vi "microspec_validating.vi"() -> ()   [LabVIEW 2009]
uses:
  <vilib>/Utility/file.llb/Write To Spreadsheet File (string).vi
  <vilib>/Instr/_visa.llb/VISA Configure Serial Port (Instr).vi
panel:
  out "error 2":dbl
  in  "Path":path
  in  "intergration time":dbl caption="sensor\nintergration time (us)" min=54.0 max=5000000.0 step=100.0
  in  "?":T1(tab)
  out "radiometer data file path":path
  in  "Runname":string
  out "Sensor_name":string
  out "Radiometer Average":dbl
  in  "Delay":dbl
  in  "Step":dbl
  in  "Stop Wl":dbl min=0.0 max=5000.0 step=100.0
  in  "Start Wl":dbl min=0.0 max=5000.0 step=100.0
  in  "mean_number":i32 caption="Mean Number"
  out "Current Wavelength":dbl
  out "XY-Graph 2":cluster{"Y":dbl[], "Y":dbl[]}[](graph)
  in  "run 5":bool
  out "sectrometer data file path":path
  in  "save data":bool
  in  "reset with every wavelength?":bool caption="reset with new run?"
  in  "Delay":dbl
  in  "Step":dbl
  in  "Stop Wl":dbl min=0.0 max=5000.0 step=100.0
  out "Current Wavelength":dbl
  in  "Start Wl 2":dbl min=0.0 max=5000.0 step=10.0
  in  "Sensor":string(combo)
  in  "run 2":bool
  in  "Set Runs":i32
  out "Current Run":i32
  in  "stop runs":bool
  out "raw_data":cluster{"Y":dbl[], "Y":dbl[]}[](graph) caption="raw data"
  out "error":dbl
  out "raw_data 2":cluster{"Y":dbl[], "Y":dbl[]}[](graph) caption="raw data"
  in  "Stopp":bool
  out "System Setup":i32
  out "DLL Version":string
  out "Get Version":i32
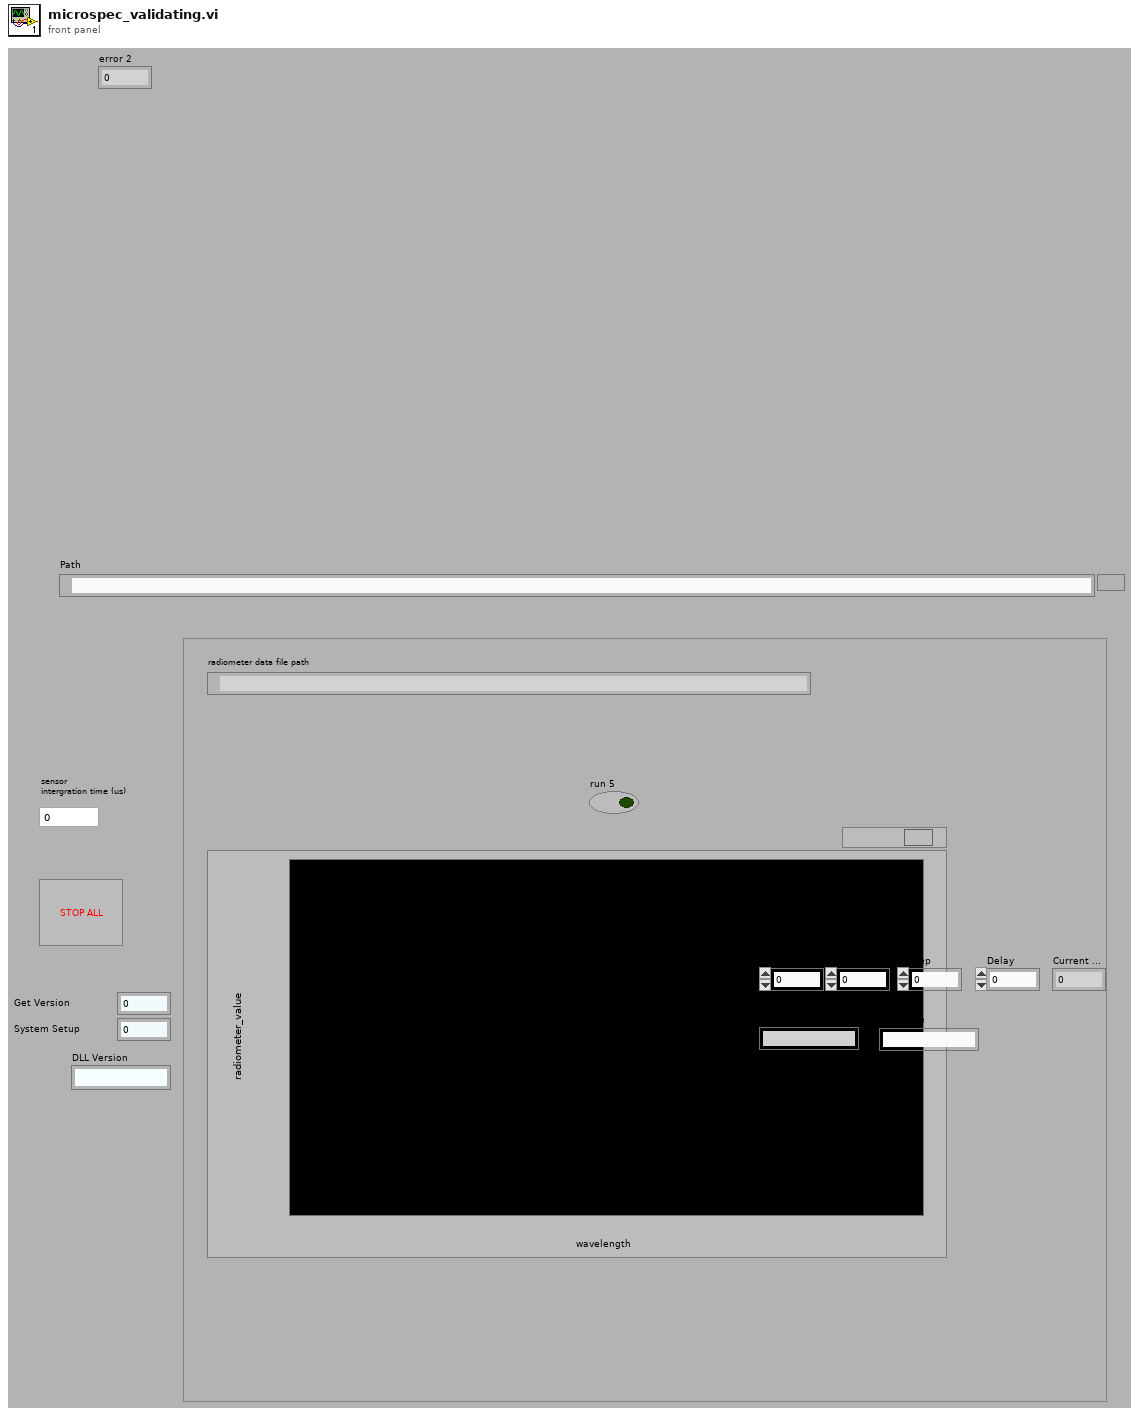
[diagram p1: front panel]
types:
  T1 = enum32{"radiometer calibration", "measuring sequence", "microspec standalone"}
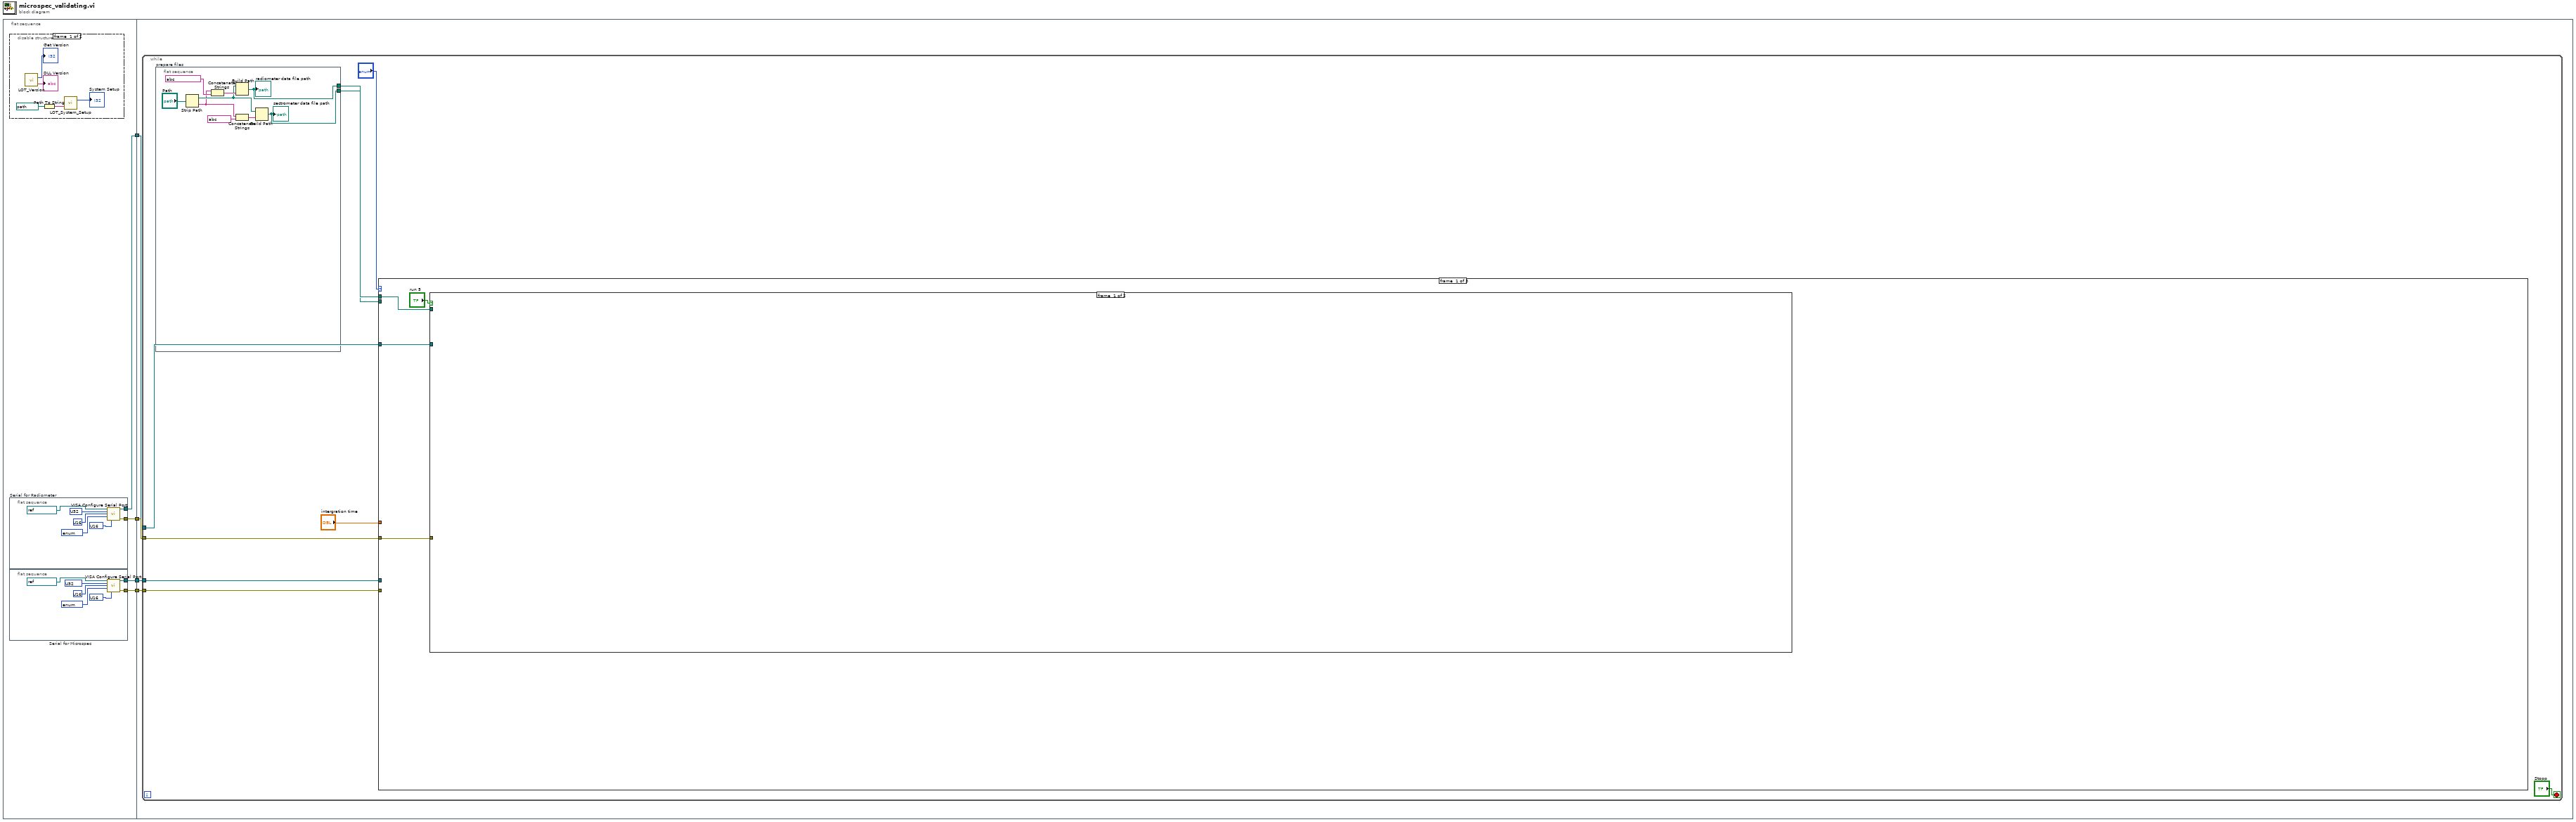
[diagram p0: block diagram]
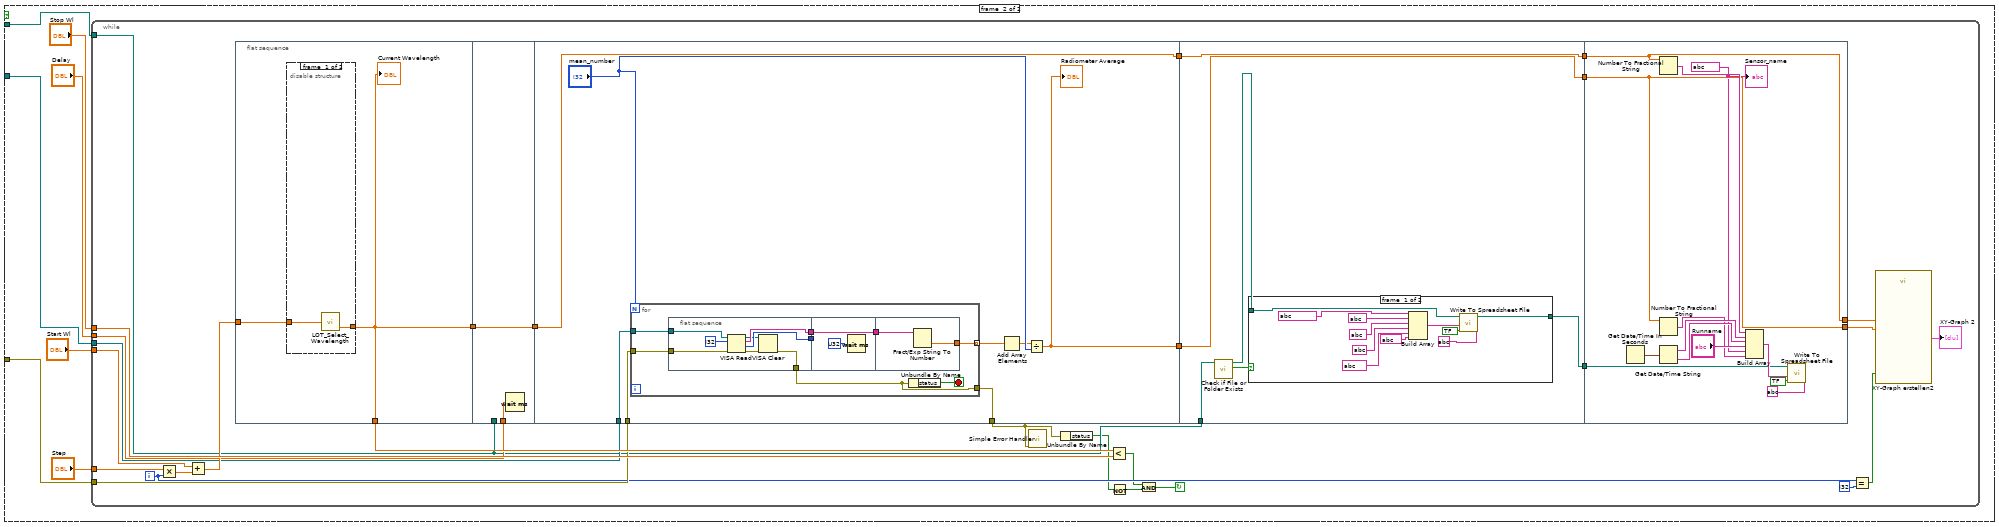
[diagram p3: hidden frame]
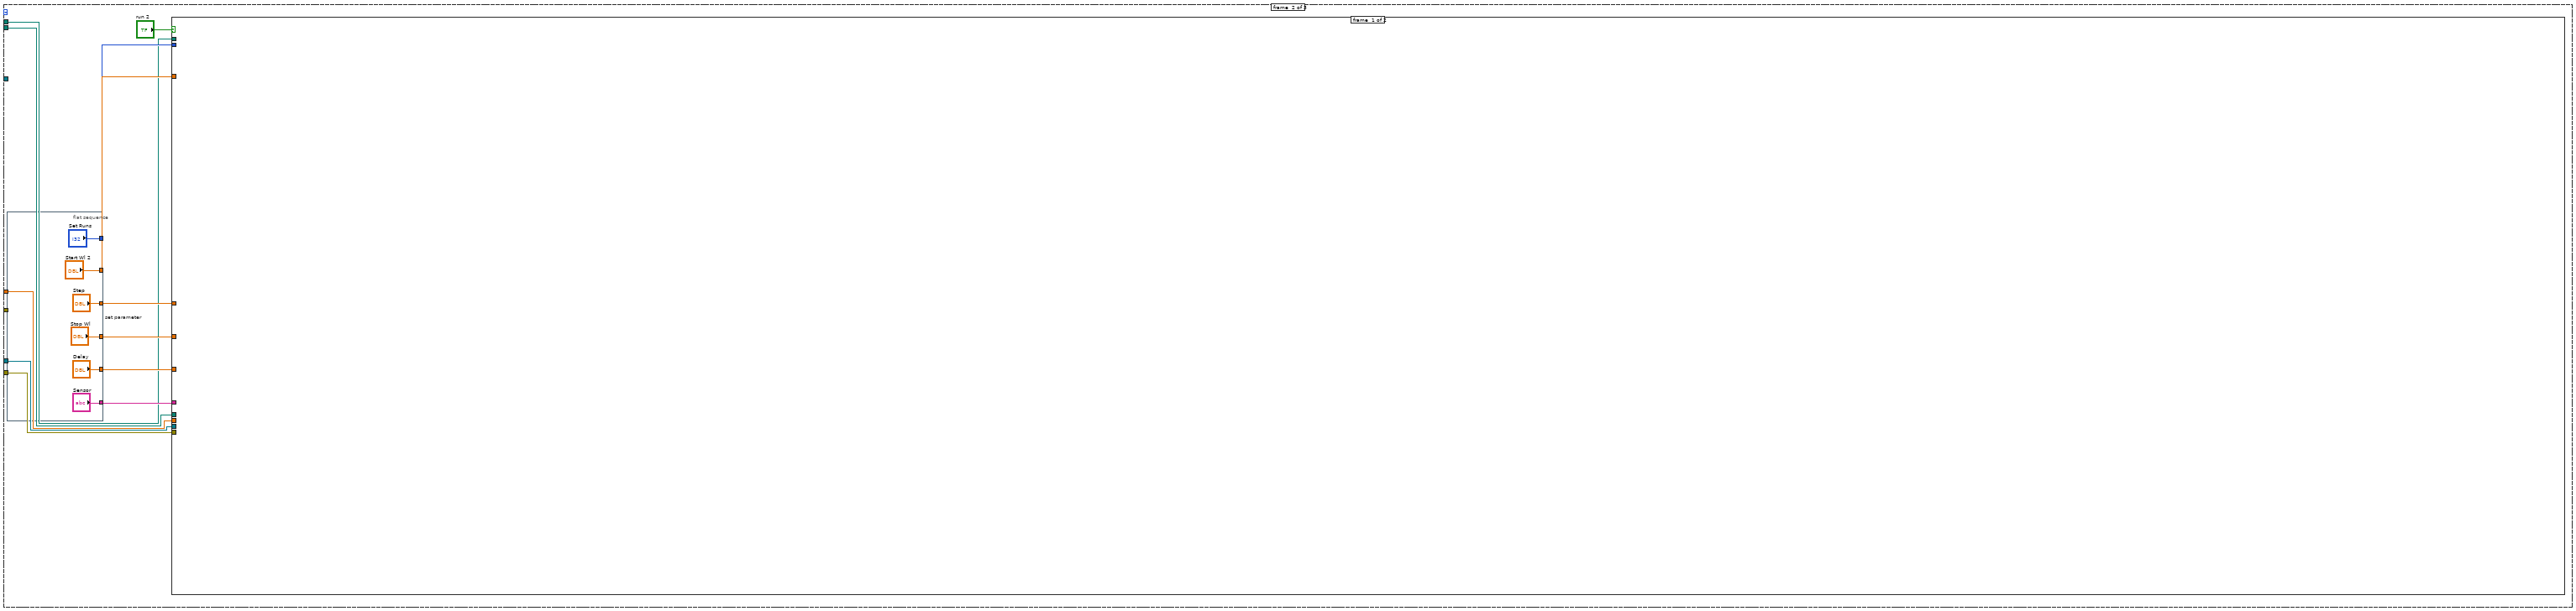
[diagram p6: hidden frame]
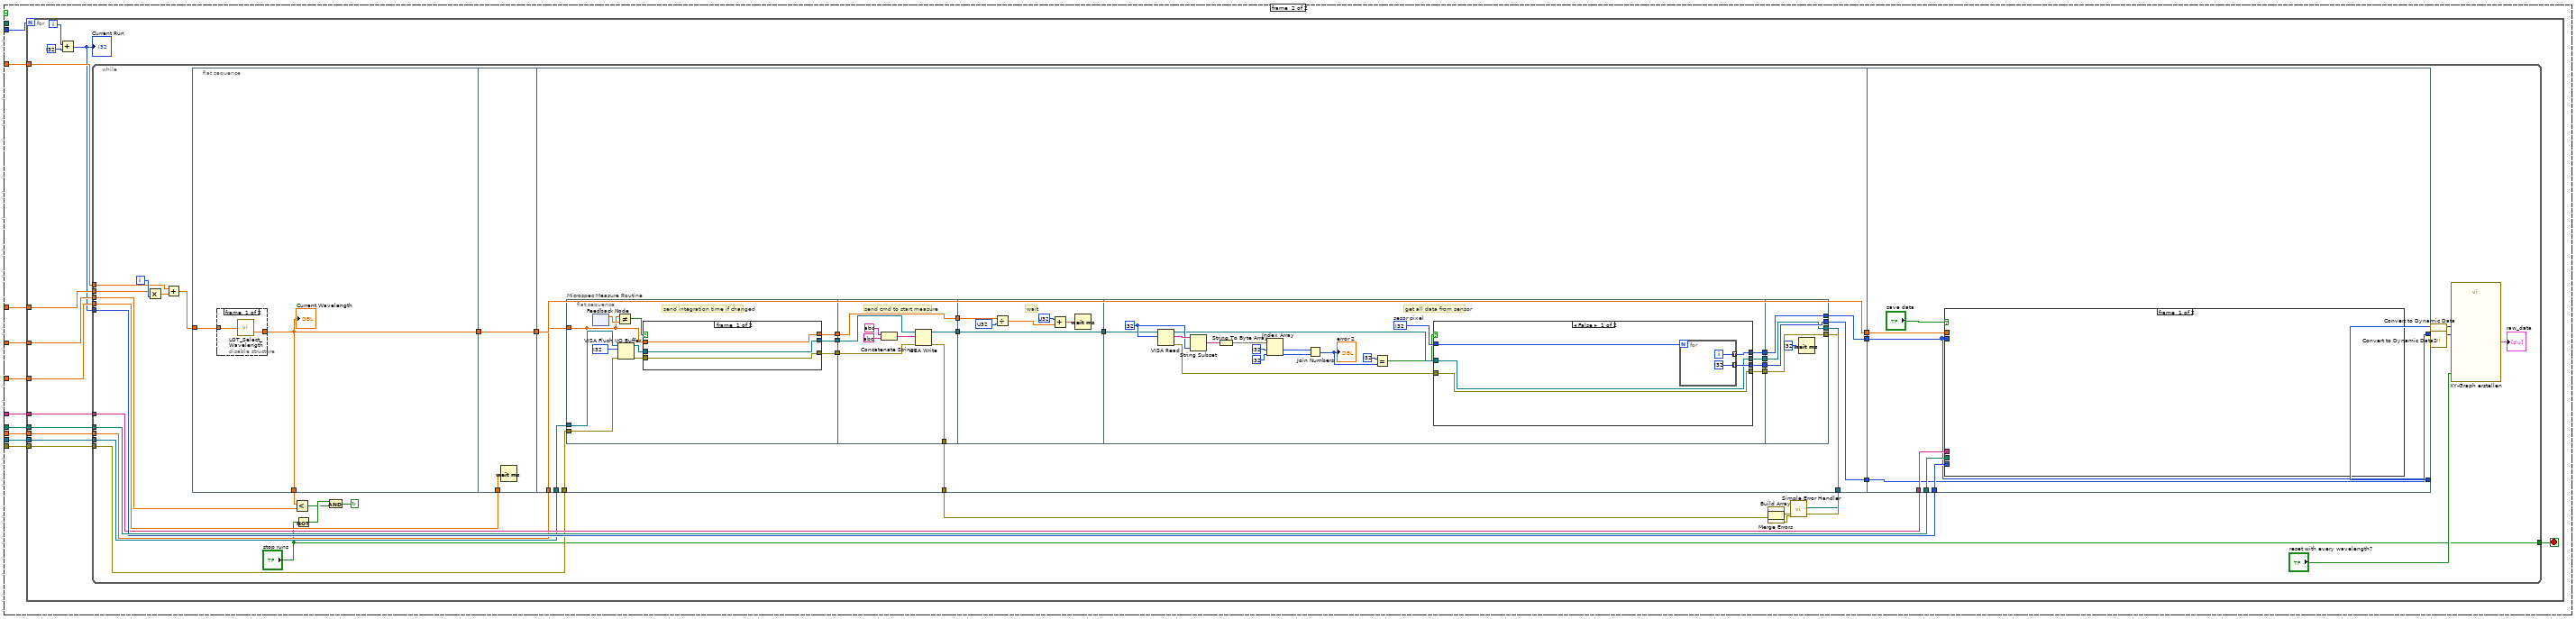
[diagram p7: hidden frame]
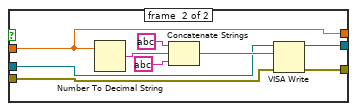
[diagram p9: hidden frame]
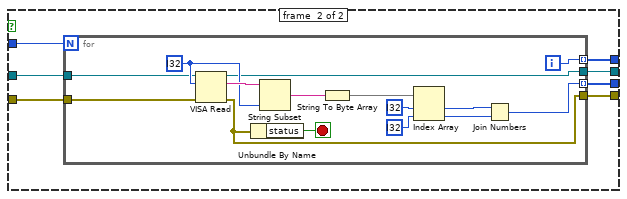
[diagram p10: hidden frame]
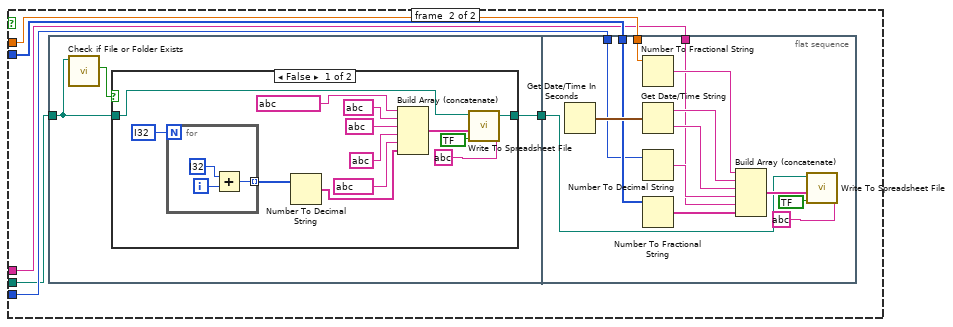
[diagram p11: hidden frame]
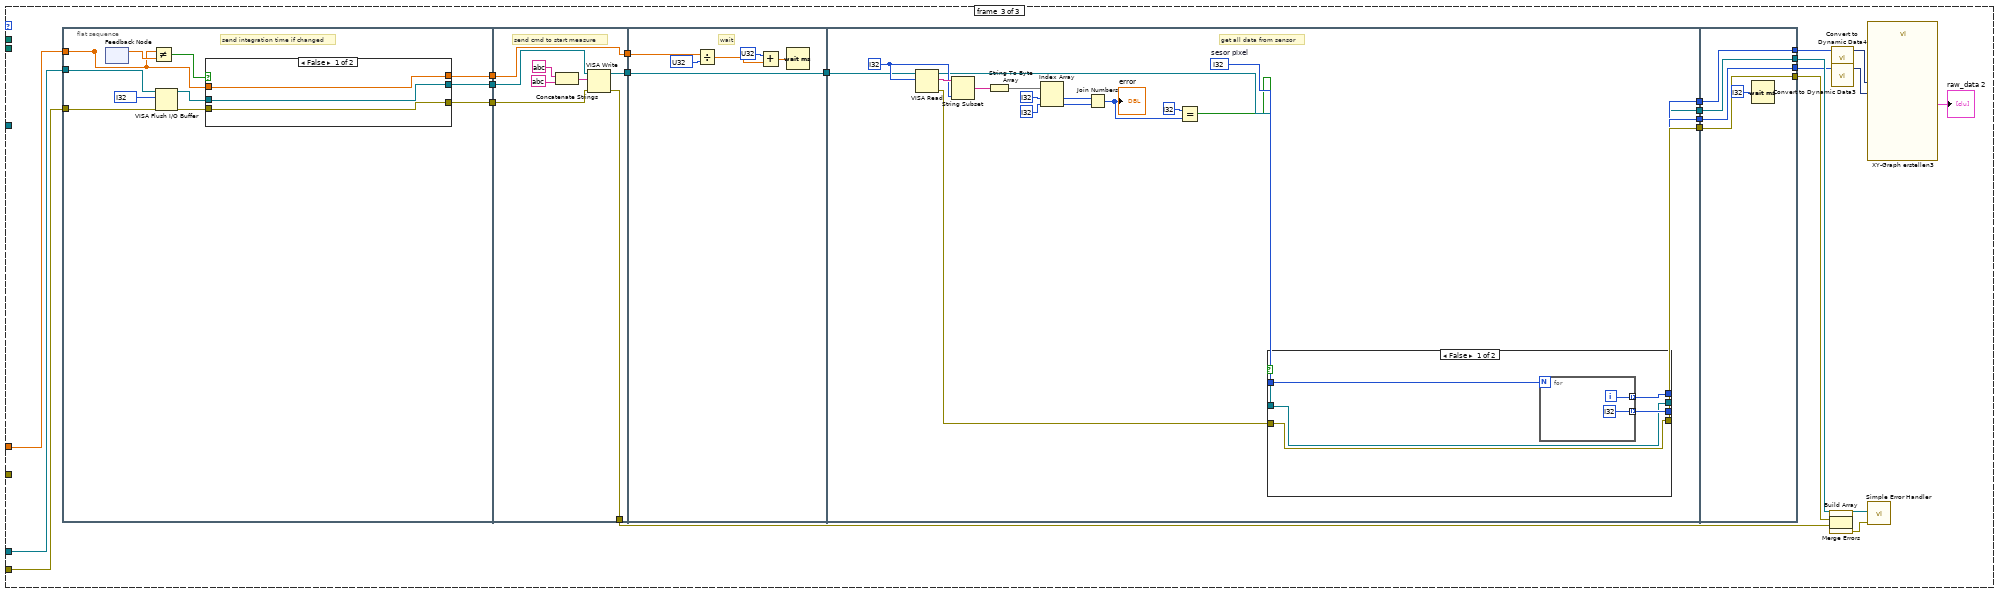
[diagram p13: hidden frame]
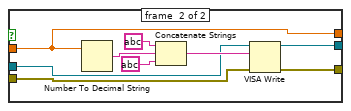
[diagram p14: hidden frame]
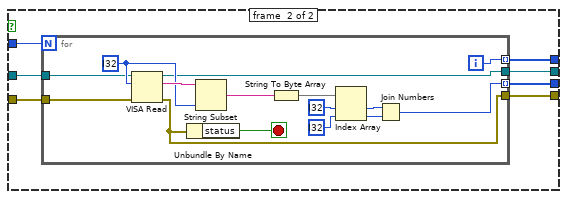
[diagram p15: hidden frame]
diagram:
  n1 = flat-sequence {
    tunnel: [w8] -> w4
    tunnel: [w7] -> w3
    tunnel: [w6] -> w2
    tunnel: [w5] -> w1
    tunnel: w4 -> [w31]
    tunnel: w3 -> [w30]
    tunnel: w2 -> [w29]
    tunnel: w1 -> [w28]
    frame #0 {
      # "Configuration"
      n2 = disable-structure shown="Enabled" {
        frame #0 {
          n3 = call "LOT_Version.vi"() -> ("Version"=→"DLL Version":string, "Get Version"=→"Get Version":i32)
          n4 = Path To String(path=path ? ("Configuration File")) -> (string=w25:string)
          n5 = call "LOT_System_Setup.vi"("CFG File Path"=w25) -> ("Error Code"=→"System Setup":i32)  [unwired: 2 in]
        }
        frame #1 {
        }
      }
      n6 = flat-sequence "Serial for Radiometer" {
        tunnel: [w15] -> w6
        tunnel: [w14] -> w5
        frame #0 {
          w10 = u16 ? items=["1.0", "1.5", "2.0"] ("stop bits (10: 1 bit)")
          n7 = call-poly "VISA Configure Serial Port"("VISA resource name"=refnum<visa-resource-name> ?, "baud rate (9600)"=u32 ?, "data bits (8)"=u16 ?, "parity (0:none)"=enum16{"None", "Odd", "Even", "Mark", "Space"} ?, "stop bits (10: 1 bit)"=w10) -> ("VISA resource name out"=w14:refnum<visa-resource-name>, "error out"=w15:errorcluster)  [unwired: 9 in]
        }
      }
      n8 = flat-sequence "Serial for Microspec" {
        tunnel: [w22] -> w8
        tunnel: [w21] -> w7
        frame #0 {
          w17 = u16 ? items=["1.0", "1.5", "2.0"] ("stop bits (10: 1 bit)")
          n9 = call-poly "VISA Configure Serial Port"("VISA resource name"=refnum<visa-resource-name> ?, "baud rate (9600)"=u32 ?, "data bits (8)"=u16 ?, "parity (0:none)"=enum16{"None", "Odd", "Even", "Mark", "Space"} ?, "stop bits (10: 1 bit)"=w17) -> ("VISA resource name out"=w22:refnum<visa-resource-name>, "error out"=w21:errorcluster)  [unwired: 9 in]
        }
      }
    }
    frame #1 {
      n10 = while {
        tunnel: w31 -> [w38]
        tunnel: w30 -> [w37]
        tunnel: w29 -> [w36]
        tunnel: w28 -> [w35]
        stop <- "Stopp" stop-if-true
        n11 = flat-sequence "prepare files" {
          tunnel: [w41] -> w32
          tunnel: [w42] -> w33
          frame #0 {
            n12 = Strip Path(path="Path") -> (stripped path=w44:path, name=w43:string)
            n13 = Concatenate Strings(w43, string ?) -> (w45:string)
            n14 = Build Path(base path=w44, name or relative path=w45) -> (appended path=w42:path)
            "radiometer data file path" <- w42
            n15 = Concatenate Strings(w43, string ?) -> (w47:string)
            n16 = Build Path(base path=w44, name or relative path=w47) -> (appended path=w41:path)
            "sectrometer data file path" <- w41
          }
        }
        n17 = case shown="\"measuring sequence\"" "?" {
          tunnel: w32 -> [_ w165 _]
          tunnel: w38 -> [_ w164 w415]
          tunnel: w37 -> [_ w163 w414]
          tunnel: w36 -> [w52 _ _]
          tunnel: w35 -> [w51 _ _]
          tunnel: "intergration time" -> [_ w162 w413]
          tunnel: w33 -> [w50 w155 _]
          frame #0 {
            n18 = case shown="True" "run 5" {
              tunnel: w50 -> [_ w56]
              tunnel: w52 -> [_ w55]
              tunnel: w51 -> [_ w54]
              frame #0 {
              }
              frame #1 {
                n19 = while {
                  tunnel: "Step" -> [w88]
                  tunnel: "Start Wl" -> [w86]
                  tunnel: "Stop Wl" -> [w85]
                  tunnel: "Delay" -> [w81]
                  tunnel: w56 -> [w67]
                  tunnel: w54 -> [w80]
                  tunnel: w55 -> [w79]
                  i -> [w75]
                  stop <- w62 continue-if-true
                  n20 = Multiply(x=w88, y=w75) -> (x*y=w87:dbl)
                  n21 = Add(x=w86, y=w87) -> (x+y=w84:dbl)
                  n22 = flat-sequence {
                    tunnel: w84 -> [w90]
                    tunnel: [w89] -> w83
                    tunnel: [w89] -> w82
                    tunnel: w67 -> [_]
                    tunnel: w82 -> [w94]
                    tunnel: w81 -> [w95]
                    tunnel: [w94] -> w78
                    tunnel: w80 -> [w103]
                    tunnel: w79 -> [w102]
                    tunnel: w78 -> [w101]
                    tunnel: [w101] -> w71
                    tunnel: [w99] -> w69
                    tunnel: [w96] -> w61
                    tunnel: w71 -> [w129]
                    tunnel: [w129] -> w70
                    tunnel: w69 -> [w128]
                    tunnel: [w128] -> w68
                    tunnel: w67 -> [w126]
                    tunnel: [w127] -> w66
                    tunnel: [w145] -> w72
                    tunnel: [w146] -> w76
                    tunnel: w70 -> [w146]
                    tunnel: w68 -> [w145]
                    tunnel: w66 -> [w148]
                    frame #0 {
                      n23 = disable-structure shown="Enabled" {
                        disable-tunnel: w90 -> [w92 w93]
                        disable-tunnel: [w91 w93] -> w89
                        frame #0 {
                          n24 = call "LOT_Select_Wavelength.vi"("Input Wavelength"=w92) -> ("Current Wavelength"=w91:dbl)  [unwired: 1 out]
                        }
                        frame #1 {
                        }
                      }
                      "Current Wavelength" <- w89
                    }
                    frame #1 {
                      n25 = Wait (ms)(milliseconds to wait=w95) -> ()  [unwired: 1 out]
                    }
                    frame #2 {
                      n26 = for {
                        N: "mean_number" -> [_]
                        tunnel: w103 -> [w108]
                        tunnel: w102 -> [w107]
                        tunnel: [w106] -> w97 mode=indexing
                        tunnel: [w105] -> w96
                        stop <- w104 stop-if-true
                        n27 = flat-sequence {
                          tunnel: [w116] -> w111
                          tunnel: w108 -> [w119]
                          tunnel: w107 -> [w118]
                          tunnel: [w115] -> w110
                          tunnel: [w112] -> w105
                          tunnel: w111 -> [w121]
                          tunnel: [w121] -> w109
                          tunnel: w110 -> [_]
                          tunnel: w109 -> [w122]
                          tunnel: [w123] -> w106
                          frame #0 {
                            n28 = VISA Read(VISA resource name=w119, byte count=i32 ?, error in (no error)=w118) -> (VISA resource name out=w113:refnum<visa-resource-name>, read buffer=w116:string, return count=w115:u32, error out=w114:errorcluster)
                            n29 = VISA Clear(VISA resource name=w113, error in (no error)=w114) -> (error out=w112:errorcluster)  [unwired: 1 out]
                          }
                          frame #1 {
                            n30 = Wait (ms)(milliseconds to wait=u32 ? ("Zu wartende ms")) -> ()  [unwired: 1 out]
                          }
                          frame #2 {
                            n31 = Fract/Exp String To Number(string=w122) -> (number=w123:dbl)  [unwired: 3 in, 1 out]
                          }
                        }
                        n32 = Unbundle By Name(w105) -> ("status"=w104:bool)
                      }
                      n33 = Add Array Elements(numeric array=w97) -> (sum=w98:dbl)
                      n34 = Divide(x=w98, y="mean_number") -> (x/y=w99:dbl)
                      "Radiometer Average" <- w99
                    }
                    frame #3 {
                      n35 = call <vilib>:"Check if File or Folder Exists.vi"("path"=w126) -> ("file or folder exists?"=w125:bool, "dup path"=w124:path)  [unwired: 8 in, 1 out]
                      n36 = case shown="True" w125 {
                        tunnel: w124 -> [w138 w141]
                        tunnel: [w131 w141] -> w127
                        frame #0 {
                          n37 = Build Array(string ?, string ? ("Element"), string ? ("Element"), string ? ("Element"), string ? ("Element"), string ?) -> (w140:string[])
                          n38 = call-poly <vilib>:"Write To Spreadsheet File.vi"("delimiter (\\t)"=string ?, "append to file? (new file:F)"=bool ?, "1D data"=w140, "file path (dialog if empty)"=w138) -> ("new file path (Not A Path if cancelled)"=w131:path)  [unwired: 4 in]
                        }
                        frame #1 {
                        }
                      }
                    }
                    frame #4 {
                      w143 = string ? ("Sensor_name")
                      n39 = Get Date/Time In Seconds() -> (seconds since 1Jan1904=w153:timestamp)
                      n40 = Number To Fractional String(number=w146) -> (F-format string=w154:string)  [unwired: 3 in]
                      n41 = Number To Fractional String(number=w145) -> (F-format string=w142:string)  [unwired: 3 in]
                      n42 = Get Date/Time String(seconds (now)=w153) -> (date string=w152:string, time string=w151:string)  [unwired: 2 in]
                      n43 = Build Array(w154, w152, w151, "Runname", w143, w142) -> (w150:string[])
                      n44 = call-poly <vilib>:"Write To Spreadsheet File.vi"("delimiter (\\t)"=string ?, "append to file? (new file:F)"=bool ?, "1D data"=w150, "file path (dialog if empty)"=w148) -> ()  [unwired: 4 in, 1 out]
                      "Sensor_name" <- w143
                    }
                  }
                  n45 = call <vilib>:"Simple Error Handler.vi"("error in (no error)"=w61) -> ()  [unwired: 4 in, 5 out]
                  n46 = Unbundle By Name(w61) -> ("status"=w63:bool)
                  n47 = Less?(x=w83, y=w85) -> (x < y?=w65:bool)
                  n48 = Not(x=w63) -> (.not. x?=w64:bool)
                  n49 = And(x=w65, y=w64) -> (x .and. y?=w62:bool)
                  n50 = Equal?(x=w75, y=i32 ?) -> (x = y?=w73:bool)
                  n51 = call "XY-Graph erstellen2"("Reset"=w73, "Y Input"=w72, "X Input"=w76) -> ("XY Graph"=→"XY-Graph 2":cluster{"Y":dbl[], "Y":dbl[]}[])  [unwired: 7 in, 1 out]
                }
              }
            }
          }
          frame #1 {
            n52 = flat-sequence "set parameter" {
              tunnel: ["Sensor"] -> w161
              tunnel: ["Delay"] -> w160
              tunnel: ["Step"] -> w159
              tunnel: ["Stop Wl"] -> w158
              tunnel: ["Start Wl 2"] -> w157
              tunnel: ["Set Runs"] -> w156
              frame #0 {
              }
            }
            n53 = case shown="True" "run 2" {
              tunnel: w165 -> [_ w173]
              tunnel: w161 -> [_ w182]
              tunnel: w156 -> [_ w181]
              tunnel: w164 -> [_ w180]
              tunnel: w163 -> [_ w179]
              tunnel: w160 -> [_ w178]
              tunnel: w158 -> [_ w177]
              tunnel: w159 -> [_ w176]
              tunnel: w157 -> [_ w175]
              tunnel: w162 -> [_ w174]
              tunnel: w155 -> [_ _]
              frame #0 {
              }
              frame #1 {
                n54 = for {
                  N: w181 -> [_]
                  tunnel: w173 -> [w195]
                  tunnel: w182 -> [w194]
                  tunnel: w180 -> [w193]
                  tunnel: w179 -> [w192]
                  tunnel: w178 -> [w191]
                  tunnel: w177 -> [w190]
                  tunnel: w176 -> [w189]
                  tunnel: w175 -> [w188]
                  tunnel: w174 -> [w187]
                  i -> [w186]
                  stop <- w183 stop-if-true
                  n55 = Add(x=w186, y=i32 ?) -> (x+y=w185:i32)
                  "Current Run" <- w185
                  n56 = while {
                    tunnel: w195 -> [w227]
                    tunnel: w185 -> [w226]
                    tunnel: w194 -> [w222]
                    tunnel: w193 -> [w220]
                    tunnel: w192 -> [w219]
                    tunnel: w191 -> [w210]
                    tunnel: w190 -> [w208]
                    tunnel: w189 -> [w207]
                    tunnel: w188 -> [w206]
                    tunnel: w187 -> [w205]
                    tunnel: ["stop runs"] -> w183
                    i -> [w224]
                    stop <- w199 continue-if-true
                    n57 = Multiply(x=w207, y=w224) -> (x*y=w229:dbl)
                    n58 = Add(x=w206, y=w229) -> (x+y=w228:dbl)
                    n59 = flat-sequence {
                      tunnel: w228 -> [w231]
                      tunnel: [w230] -> w225
                      tunnel: [w230] -> w209
                      tunnel: w225 -> [w235]
                      tunnel: w210 -> [w236]
                      tunnel: [w235] -> w213
                      tunnel: [w244] -> w221
                      tunnel: w220 -> [w248]
                      tunnel: w219 -> [w249]
                      tunnel: [w247] -> w217
                      tunnel: [w246] -> w216
                      tunnel: [w245] -> w215
                      tunnel: w213 -> [w244]
                      tunnel: w205 -> [w243]
                      tunnel: [w242] -> w204
                      tunnel: [w241] -> w197
                      tunnel: w227 -> [w352]
                      tunnel: w221 -> [w351]
                      tunnel: w226 -> [w350]
                      tunnel: [w348] -> w211
                      tunnel: w222 -> [w349]
                      tunnel: w215 -> [w348]
                      tunnel: w204 -> [w347]
                      tunnel: [w347] -> w203
                      frame #0 {
                        # "set wavelength"
                        n60 = disable-structure shown="Enabled" {
                          disable-tunnel: w231 -> [w233 w234]
                          disable-tunnel: [w232 w234] -> w230
                          frame #0 {
                            n61 = call "LOT_Select_Wavelength.vi"("Input Wavelength"=w233) -> ("Current Wavelength"=w232:dbl)  [unwired: 1 out]
                          }
                          frame #1 {
                          }
                        }
                        "Current Wavelength" <- w230
                      }
                      frame #1 {
                        # "wait"
                        n62 = Wait (ms)(milliseconds to wait=w236) -> ()  [unwired: 1 out]
                      }
                      frame #2 {
                        n63 = flat-sequence "Microspec Measure Routine" {
                          tunnel: w248 -> [w257]
                          tunnel: w249 -> [w266]
                          tunnel: [w261] -> w255
                          tunnel: [w260] -> w254
                          tunnel: [w259] -> w253
                          tunnel: w243 -> [w256]
                          tunnel: [w283] -> w252
                          tunnel: [w282] -> w246
                          tunnel: w255 -> [w280]
                          tunnel: w254 -> [w281]
                          tunnel: w253 -> [w279]
                          tunnel: [w279] -> w251
                          tunnel: w252 -> [w288]
                          tunnel: [w288] -> w250
                          tunnel: w251 -> [w287]
                          tunnel: w250 -> [w297]
                          tunnel: [w296] -> w240
                          tunnel: [w295] -> w239
                          tunnel: [w294] -> w238
                          tunnel: [w293] -> w237
                          tunnel: [w342] -> w241
                          tunnel: [w343] -> w247
                          tunnel: [w344] -> w242
                          tunnel: [w345] -> w245
                          tunnel: w240 -> [w345]
                          tunnel: w239 -> [w344]
                          tunnel: w238 -> [w343]
                          tunnel: w237 -> [w342]
                          frame #0 {
                            # "send integration time if changed"
                            n64 = feedback #1() -> (w265:dbl)  [unwired: 1 in]
                            n65 = Not Equal?(x=w256, y=w265) -> (x != y?=w264:bool)
                            n66 = VISA Flush I/O Buffer(VISA resource name=w257, mask (16)=i32 ?, error in (no error)=w266) -> (VISA resource name out=w263:refnum<visa-resource-name>, error out=w262:errorcluster)
                            n67 = case shown="True" w264 {
                              tunnel: w263 -> [w268 w274]
                              tunnel: w262 -> [w267 w273]
                              tunnel: [w267 w272] -> w261
                              tunnel: [w268 w271] -> w260
                              tunnel: w256 -> [w269 w270]
                              tunnel: [w269 w270] -> w259
                              frame #0 {
                              }
                              frame #1 {
                                n68 = Number To Decimal String(number=w270) -> (decimal integer string=w277:string)  [unwired: 1 in]
                                n69 = Concatenate Strings(string ?, w277, string ?) -> (w275:string)
                                n70 = VISA Write(VISA resource name=w274, write buffer=w275, error in (no error)=w273) -> (VISA resource name out=w271:refnum<visa-resource-name>, error out=w272:errorcluster)  [unwired: 1 out]
                              }
                            }
                          }
                          frame #1 {
                            # "send cmd to start measure"
                            n71 = Concatenate Strings(string ?, string ?) -> (w284:string)
                            n72 = VISA Write(VISA resource name=w281, write buffer=w284, error in (no error)=w280) -> (VISA resource name out=w283:refnum<visa-resource-name>, error out=w282:errorcluster)  [unwired: 1 out]
                          }
                          frame #2 {
                            # "wait"
                            n73 = Divide(x=w287, y=u32 ? ("Zu wartende ms")) -> (x/y=w289:dbl)
                            n74 = Add(x=u32 ? ("Zu wartende ms"), y=w289) -> (x+y=w291:dbl)
                            n75 = Wait (ms)(milliseconds to wait=w291) -> ()  [unwired: 1 out]
                          }
                          frame #3 {
                            w309 = i32 ?
                            w311 = i32 ?  # sesor pixel
                            # "get all data from sensor"
                            n76 = VISA Read(VISA resource name=w297, byte count=w309) -> (VISA resource name out=w302:refnum<visa-resource-name>, read buffer=w310:string, error out=w299:errorcluster)  [unwired: 1 in, 1 out]
                            n77 = String Subset(string=w310, length (rest)=w309) -> (substring=w308:string)  [unwired: 1 in]
                            n78 = String To Byte Array(string=w308) -> (unsigned byte array=w307:u8[])
                            n79 = Index Array(array=w307, index #1=i32 ?, index #2=i32 ?) -> (element #1=w303:u8, element #2=w304:u8)
                            n80 = Join Numbers(hi=w303, lo=w304) -> ((hi.lo)=w300:u16)
                            "error 2" <- w300
                            n81 = Equal?(x=i32 ?, y=w300) -> (x = y?=w298:bool)
                            n82 = case shown="False" w298 {
                              tunnel: [w314 w325] -> w294
                              tunnel: w302 -> [w313 w324]
                              tunnel: [w315 w323] -> w295
                              tunnel: [w316 w322] -> w296
                              tunnel: w311 -> [w312 w321]
                              tunnel: [w313 w320] -> w293
                              tunnel: w299 -> [w314 w319]
                              frame #0 {
                                n83 = for {
                                N: w312 -> [_]
                                tunnel: [i32 ?] -> w315 mode=indexing
                                tunnel: [w318] -> w316 mode=indexing
                                i -> [w318]
                                }
                              }
                              frame #1 {
                                n84 = for {
                                N: w321 -> [_]
                                tunnel: w324 -> [w330]
                                tunnel: [w329] -> w325
                                tunnel: [w332] -> w323 mode=indexing
                                tunnel: [w331] -> w322 mode=indexing
                                tunnel: [w327] -> w320
                                tunnel: w319 -> [w326]
                                i -> [w331]
                                stop <- w328 stop-if-true
                                w339 = i32 ?
                                n85 = VISA Read(VISA resource name=w330, byte count=w339, error in (no error)=w326) -> (VISA resource name out=w327:refnum<visa-resource-name>, read buffer=w340:string, error out=w329:errorcluster)  [unwired: 1 out]
                                n86 = Unbundle By Name(w329) -> ("status"=w328:bool)
                                n87 = String Subset(string=w340, length (rest)=w339) -> (substring=w338:string)  [unwired: 1 in]
                                n88 = String To Byte Array(string=w338) -> (unsigned byte array=w337:u8[])
                                n89 = Index Array(array=w337, index #1=i32 ?, index #2=i32 ?) -> (element #1=w333:u8, element #2=w334:u8)
                                n90 = Join Numbers(hi=w333, lo=w334) -> ((hi.lo)=w332:u16)
                                }
                              }
                            }
                          }
                          frame #4 {
                            n91 = Wait (ms)(milliseconds to wait=i32 ?) -> ()  [unwired: 1 out]
                          }
                        }
                      }
                      frame #3 {
                        n92 = case shown="True" "save data" {
                          tunnel: w352 -> [_ w355]
                          tunnel: w351 -> [_ w357]
                          tunnel: w350 -> [_ w356]
                          tunnel: w348 -> [_ w358]
                          tunnel: w349 -> [_ w354]
                          frame #0 {
                          }
                          frame #1 {
                            n93 = flat-sequence {
                              tunnel: w355 -> [w361]
                              tunnel: [w359] -> w353
                              tunnel: w358 -> [w385]
                              tunnel: w357 -> [w384]
                              tunnel: w356 -> [w383]
                              tunnel: w354 -> [w381]
                              tunnel: w353 -> [w379]
                              frame #0 {
                                n94 = call <vilib>:"Check if File or Folder Exists.vi"("path"=w361) -> ("file or folder exists?"=w360:bool)  [unwired: 8 in, 2 out]
                                n95 = case shown="False" w360 {
                                tunnel: w361 -> [w365 w378]
                                tunnel: [w362 w378] -> w359
                                frame #0 {
                                n96 = for {
                                N: i32 ? -> [_]
                                tunnel: [w375] -> w368 mode=indexing
                                i -> [w377]
                                n97 = Add(x=i32 ?, y=w377) -> (x+y=w375:i32)
                                }
                                n98 = Number To Decimal String(number=w368) -> (decimal integer string=w370:string[])  [unwired: 1 in]
                                n99 = Build Array (concatenate)(string ?, string ? ("Element"), string ? ("Element"), string ? ("Element"), string ? ("Element"), w370) -> (w374:string[])
                                n100 = call-poly <vilib>:"Write To Spreadsheet File.vi"("delimiter (\\t)"=string ?, "append to file? (new file:F)"=bool ?, "1D data"=w374, "file path (dialog if empty)"=w365) -> ("new file path (Not A Path if cancelled)"=w362:path)  [unwired: 4 in]
                                }
                                frame #1 {
                                }
                                }
                              }
                              frame #1 {
                                n101 = Get Date/Time In Seconds() -> (seconds since 1Jan1904=w387:timestamp)
                                n102 = Number To Fractional String(number=w384) -> (F-format string=w386:string)  [unwired: 3 in]
                                n103 = Get Date/Time String(seconds (now)=w387) -> (date string=w388:string, time string=w389:string)  [unwired: 2 in]
                                n104 = Number To Decimal String(number=w383) -> (decimal integer string=w382:string)  [unwired: 1 in]
                                n105 = Number To Fractional String(number=w385) -> (F-format string=w392:string[])  [unwired: 3 in]
                                n106 = Build Array (concatenate)(w386, w388, w389, w382, w381, w392) -> (w390:string[])
                                n107 = call-poly <vilib>:"Write To Spreadsheet File.vi"("delimiter (\\t)"=string ?, "append to file? (new file:F)"=bool ?, "1D data"=w390, "file path (dialog if empty)"=w379) -> ()  [unwired: 4 in, 1 out]
                              }
                            }
                          }
                        }
                      }
                    }
                    n108 = Less?(x=w209, y=w208) -> (x < y?=w200:bool)
                    n109 = Not(x="stop runs") -> (.not. x?=w201:bool)
                    n110 = And(x=w201, y=w200) -> (x .and. y?=w199:bool)
                    n111 = Build Array(w217, w216) -> (w196:errorcluster[])
                    n112 = call <vilib>:"Merge Errors.vi"("error array in"=w196) -> ("error out"=w218:errorcluster)  [unwired: 6 in]
                    n113 = call <vilib>:"Simple Error Handler.vi"("error source (\" \")"=w197, "error in (no error)"=w218) -> ()  [unwired: 3 in, 5 out]
                    n114 = call "Convert to Dynamic Data"("Array"=w203) -> ("Dynamic Data Type"=w212:dynamicdata)  [unwired: 3 in]
                    n115 = call "Convert to Dynamic Data2"("Array"=w211) -> ("Dynamic Data Type"=w214:dynamicdata)  [unwired: 3 in]
                    n116 = call "XY-Graph erstellen"("Reset"="reset with every wavelength?", "Y Input"=w214, "X Input"=w212) -> ("XY Graph"=→"raw_data":cluster{"Y":dbl[], "Y":dbl[]}[])  [unwired: 7 in, 1 out]
                  }
                }
              }
            }
          }
          frame #2 {
            n117 = flat-sequence {
              tunnel: w415 -> [w425]
              tunnel: w414 -> [w426]
              tunnel: [w420] -> w412
              tunnel: [w419] -> w411
              tunnel: [w418] -> w410
              tunnel: w413 -> [w416]
              tunnel: [w443] -> w409
              tunnel: [w442] -> w405
              tunnel: w412 -> [w440]
              tunnel: w411 -> [w441]
              tunnel: w410 -> [w439]
              tunnel: [w439] -> w408
              tunnel: w409 -> [w448]
              tunnel: [w448] -> w407
              tunnel: w408 -> [w447]
              tunnel: w407 -> [w458]
              tunnel: [w471] -> w397
              tunnel: [w470] -> w396
              tunnel: [w469] -> w395
              tunnel: [w467] -> w394
              tunnel: [w502] -> w403
              tunnel: [w503] -> w398
              tunnel: [w504] -> w399
              tunnel: [w505] -> w406
              tunnel: w397 -> [w505]
              tunnel: w396 -> [w504]
              tunnel: w395 -> [w503]
              tunnel: w394 -> [w502]
              frame #0 {
                # "send integration time if changed"
                n118 = feedback #2() -> (w424:dbl)  [unwired: 1 in]
                n119 = Not Equal?(x=w416, y=w424) -> (x != y?=w423:bool)
                n120 = VISA Flush I/O Buffer(VISA resource name=w425, mask (16)=i32 ?, error in (no error)=w426) -> (VISA resource name out=w422:refnum<visa-resource-name>, error out=w421:errorcluster)
                n121 = case shown="False" w423 {
                  tunnel: w422 -> [w428 w434]
                  tunnel: w421 -> [w427 w433]
                  tunnel: [w427 w432] -> w420
                  tunnel: [w428 w431] -> w419
                  tunnel: w416 -> [w429 w430]
                  tunnel: [w429 w430] -> w418
                  frame #0 {
                  }
                  frame #1 {
                    n122 = Number To Decimal String(number=w430) -> (decimal integer string=w437:string)  [unwired: 1 in]
                    n123 = Concatenate Strings(string ?, w437, string ?) -> (w435:string)
                    n124 = VISA Write(VISA resource name=w434, write buffer=w435, error in (no error)=w433) -> (VISA resource name out=w431:refnum<visa-resource-name>, error out=w432:errorcluster)  [unwired: 1 out]
                  }
                }
              }
              frame #1 {
                # "send cmd to start measure"
                n125 = Concatenate Strings(string ?, string ?) -> (w444:string)
                n126 = VISA Write(VISA resource name=w441, write buffer=w444, error in (no error)=w440) -> (VISA resource name out=w443:refnum<visa-resource-name>, error out=w442:errorcluster)  [unwired: 1 out]
              }
              frame #2 {
                # "wait"
                n127 = Divide(x=w447, y=u32 ? ("Zu wartende ms")) -> (x/y=w449:dbl)
                n128 = Add(x=u32 ? ("Zu wartende ms"), y=w449) -> (x+y=w451:dbl)
                n129 = Wait (ms)(milliseconds to wait=w451) -> ()  [unwired: 1 out]
              }
              frame #3 {
                w465 = i32 ?
                w468 = i32 ?  # sesor pixel
                # "get all data from sensor"
                n130 = VISA Read(VISA resource name=w458, byte count=w465) -> (VISA resource name out=w457:refnum<visa-resource-name>, read buffer=w466:string, error out=w454:errorcluster)  [unwired: 1 in, 1 out]
                n131 = String Subset(string=w466, length (rest)=w465) -> (substring=w464:string)  [unwired: 1 in]
                n132 = String To Byte Array(string=w464) -> (unsigned byte array=w463:u8[])
                n133 = Index Array(array=w463, index #1=i32 ?, index #2=i32 ?) -> (element #1=w459:u8, element #2=w460:u8)
                n134 = Join Numbers(hi=w459, lo=w460) -> ((hi.lo)=w455:u16)
                "error" <- w455
                n135 = Equal?(x=i32 ?, y=w455) -> (x = y?=w453:bool)
                n136 = case shown="False" w453 {
                  tunnel: [w474 w485] -> w471
                  tunnel: w457 -> [w473 w484]
                  tunnel: [w475 w483] -> w470
                  tunnel: [w476 w482] -> w469
                  tunnel: w468 -> [w472 w481]
                  tunnel: [w473 w480] -> w467
                  tunnel: w454 -> [w474 w479]
                  frame #0 {
                    n137 = for {
                      N: w472 -> [_]
                      tunnel: [i32 ?] -> w475 mode=indexing
                      tunnel: [w478] -> w476 mode=indexing
                      i -> [w478]
                    }
                  }
                  frame #1 {
                    n138 = for {
                      N: w481 -> [_]
                      tunnel: w484 -> [w490]
                      tunnel: [w489] -> w485
                      tunnel: [w492] -> w483 mode=indexing
                      tunnel: [w491] -> w482 mode=indexing
                      tunnel: [w487] -> w480
                      tunnel: w479 -> [w486]
                      i -> [w491]
                      stop <- w488 stop-if-true
                      w499 = i32 ?
                      n139 = VISA Read(VISA resource name=w490, byte count=w499, error in (no error)=w486) -> (VISA resource name out=w487:refnum<visa-resource-name>, read buffer=w500:string, error out=w489:errorcluster)  [unwired: 1 out]
                      n140 = Unbundle By Name(w489) -> ("status"=w488:bool)
                      n141 = String Subset(string=w500, length (rest)=w499) -> (substring=w498:string)  [unwired: 1 in]
                      n142 = String To Byte Array(string=w498) -> (unsigned byte array=w497:u8[])
                      n143 = Index Array(array=w497, index #1=i32 ?, index #2=i32 ?) -> (element #1=w493:u8, element #2=w494:u8)
                      n144 = Join Numbers(hi=w493, lo=w494) -> ((hi.lo)=w492:u16)
                    }
                  }
                }
              }
              frame #4 {
                n145 = Wait (ms)(milliseconds to wait=i32 ?) -> ()  [unwired: 1 out]
              }
            }
            n146 = Build Array(w406, w405) -> (w393:errorcluster[])
            n147 = call <vilib>:"Merge Errors.vi"("error array in"=w393) -> ("error out"=w404:errorcluster)  [unwired: 6 in]
            n148 = call "Convert to Dynamic Data4"("Array"=w398) -> ("Dynamic Data Type"=w400:dynamicdata)  [unwired: 3 in]
            n149 = call "Convert to Dynamic Data3"("Array"=w399) -> ("Dynamic Data Type"=w401:dynamicdata)  [unwired: 3 in]
            n150 = call "XY-Graph erstellen3"("Y Input"=w401, "X Input"=w400) -> ("XY Graph"=→"raw_data 2":cluster{"Y":dbl[], "Y":dbl[]}[])  [unwired: 8 in, 1 out]
            n151 = call <vilib>:"Simple Error Handler.vi"("error source (\" \")"=w403, "error in (no error)"=w404) -> ()  [unwired: 3 in, 5 out]
          }
        }
      }
    }
  }
